vi "Serialize - Text.vi"(8 "error in":errorcluster, 11 "PAS Cell Data in":refnum<class "PAS Cell Data.lvclass">) -> (0 "error out":errorcluster, 2 "Serialized Text":string, 3 "PAS Cell Data out":refnum<class "PAS Cell Data.lvclass">)   [LabVIEW 2014, in "PAS Library.lvlib" / "PAS Cell Data.lvclass"]
uses:
  PAS Cell Data.lvclass
  PAS Cell Data.lvclass/PAS Cell Data.ctl
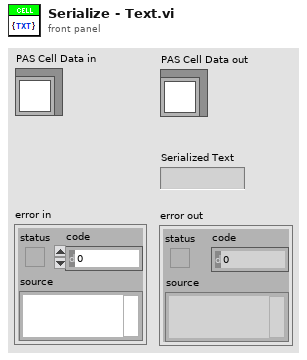
[diagram p1: front panel]
types:
  T1 = cluster{"f0":sgl, "IA":sgl, "Q":sgl, "max":dbl[], "noiseLim":dbl, "abs":dbl}
  T2 = typedef "NI_Matrix.lvlib/RealMatrix.ctl" = dbl[][]
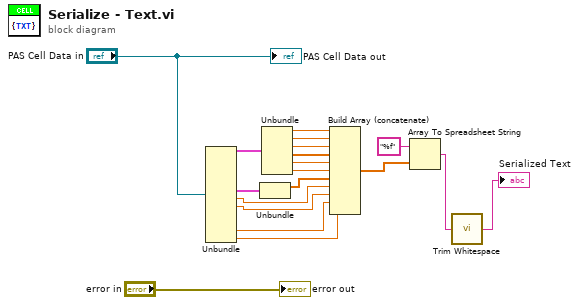
[diagram p0: block diagram]
diagram:
  n1 = Unbundle("PAS Cell Data in") -> (w16:T1, w17:cluster{"parameters":dbl[], "covariance":T2}, w8:dbl, w7:dbl, w2:dbl, w1:dbl)  [unwired: 6 out]
  n2 = Unbundle(w17) -> ("parameters"=w9:dbl[])  [unwired: 1 out]
  n3 = Unbundle(w16) -> ("f0"=w15:sgl, "IA"=w14:sgl, "Q"=w13:sgl, "max"=w12:dbl[], "noiseLim"=w11:dbl, "abs"=w10:dbl)
  n4 = Build Array (concatenate)(w15, w14, w13, w12, w11, w10, w9, w8, w7, w2, w1) -> (w6:dbl[])
  n5 = Array To Spreadsheet String(array=w6, 3:"%f" ("format string")) -> (spreadsheet string=w4:string)  [unwired: 1 in]
  n6 = call <vilib>:"Trim Whitespace.vi"("string"=w4) -> ("trimmed string"=→"Serialized Text":string)  [unwired: 1 in]
  "error out" <- "error in"
  "PAS Cell Data out" <- "PAS Cell Data in"
